vi "Set Data in Buffer.vi"(8 "error in (no error)":errorcluster, 9 "t0":timestamp, 10 "Data in":dbl[](array[numeric]), 11 "Buffer Data in":T1) -> (0 "error out":errorcluster, 1 "Buffer Full":bool, 3 "Buffer Data out":T1)   [LabVIEW 2015, in "Triggered Log.lvclass"]
uses:
  Triggered Log.lvclass
  Buffer Data.ctl
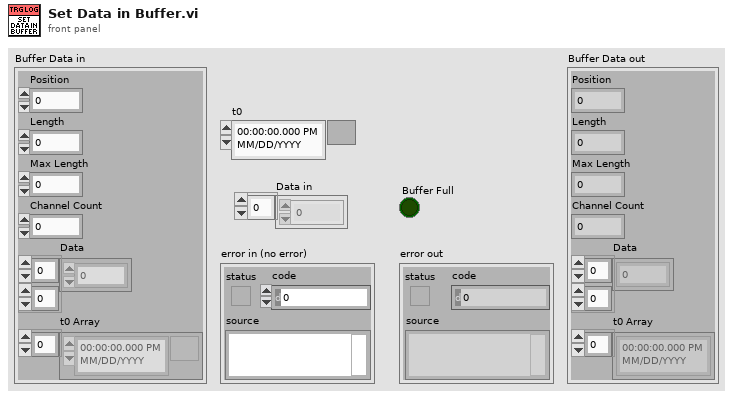
[diagram p1: front panel]
types:
  T1 = typedef "Triggered Log.lvclass/Buffer Data.ctl" = cluster{"Position":i32, "Length":i32, "Max Length":i32, "Channel Count":i32, "Data":dbl[][], "t0 Array":timestamp[]}
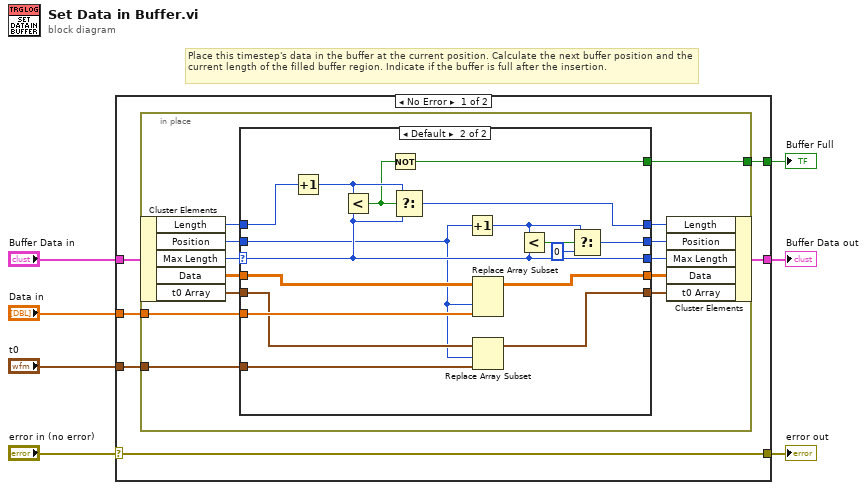
[diagram p0: block diagram]
diagram:
  # "Place this timestep's data in the buffer at the current position. Calculate the next buffer position and the current length of the filled buffer region. Indicate if the buffer is full after the insertion."
  n1 = case shown="No Error" "error in (no error)" {
    selector: "error in (no error)" -> [w9 w50]
    tunnel: [w13 w49] -> w7
    tunnel: "Buffer Data in" -> [w12 w49]
    tunnel: [w11 _] -> w5
    tunnel: "Data in" -> [w10 _]
    tunnel: [w9 w50] -> w2
    tunnel: "t0" -> [w8 _]
    frame No Error {
      n2 = in-place {
        in-place-border: w10 -> [w19]
        in-place-border: [w25] -> w11
        in-place-border: w8 -> [w14]
        n3 = in-place-cluster #1(w12) -> ("Length"=w21:i32, "Position"=w24:i32, "Max Length"=w18:i32, "Data"=w26:dbl[][], "t0 Array"=w16:timestamp[])
        n4 = case shown="Default" w18 {
          selector: w18 -> [w31 w48]
          tunnel: w26 -> [w28 w47]
          tunnel: [_ w42] -> w25
          tunnel: w24 -> [w29 w34]
          tunnel: [w29 w38] -> w23
          tunnel: [w28 w46] -> w22
          tunnel: w21 -> [w30 w44]
          tunnel: [w30 w41] -> w20
          tunnel: w19 -> [_ w45]
          tunnel: [w31 w48] -> w17
          tunnel: w16 -> [w27 w35]
          tunnel: [w27 w33] -> w15
          tunnel: w14 -> [_ w32]
          frame 0 {
            # "Empty buffer. Do nothing."
          }
          frame Default {
            n5 = Increment(x=w44) -> (x+1=w43:i32)
            n6 = Less?(x=w43, y=w48) -> (x < y?=w36:bool)
            n7 = Not(x=w36) -> (.not. x?=w42:bool)
            n8 = Select(t=w43, s=w36, f=w48) -> (s? t:f=w41:i32)
            n9 = Increment(x=w34) -> (x+1=w39:i32)
            n10 = Replace Array Subset(array=w47, new element=w45, index (col)=w34) -> (w46:dbl[][])  [unwired: 1 in]
            n11 = Replace Array Subset(array=w35, new element=w32, index=w34) -> (w33:timestamp[])
            n12 = Less?(x=w39, y=w48) -> (x < y?=w40:bool)
            n13 = Select(t=w39, s=w40, f=0) -> (s? t:f=w38:i32)
          }
        }
        n14 = in-place-cluster #1("Length"=w20, "Position"=w23, "Max Length"=w17, "Data"=w22, "t0 Array"=w15) -> (w13:T1)
      }
    }
    frame Error {
    }
  }
  "Buffer Data out" <- w7
  "Buffer Full" <- w5
  "error out" <- w2
